vi "g_tabSetting.vi"() -> ()   [LabVIEW 2015, in "ActorManagement.lvlib"]
uses:
  actorManagement/ActorManagement.lvlib
panel:
  in  "NumsInOnePage":u32=10 max=10
  in  "DeafaultBackgoundColor":u32(colorbox)=42751
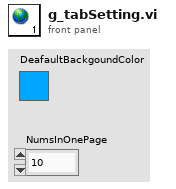
[diagram p1: front panel]
diagram:
